vi "Read Theme.vi"(8 "error in":errorcluster, 11 "Popup in":refnum<class "Popup.lvclass">) -> (0 "error out":errorcluster, 2 "Theme.lvclass":refnum<class "Theme.lvclass">, 3 "Popup out":refnum<class "Popup.lvclass">)   [LabVIEW 2021, in "Pop-Up.lvlib" / "Popup.lvclass"]
doc: "Read the theme of the pop up\n\n<b>Code Developed By:</b> +\nDaniel Coons +\nhttps://github.com/danielcoons/tsc-pop-up"
uses:
  Popup.lvclass
  Theme/Theme.lvclass
  Popup.lvclass/Popup.ctl
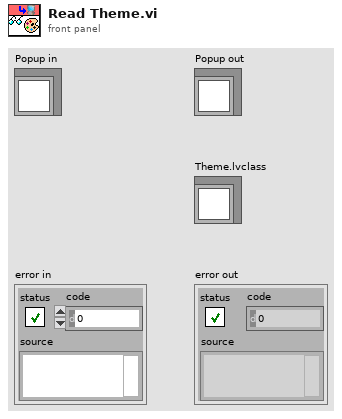
[diagram p1: front panel]
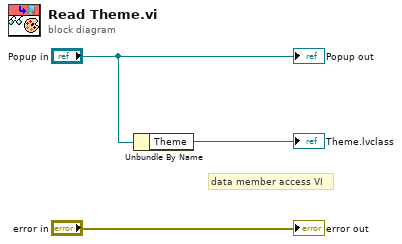
[diagram p0: block diagram]
diagram:
  # "data member access VI"
  n1 = Unbundle By Name("Popup in") -> ("Theme"=→"Theme.lvclass":refnum<class "Theme.lvclass">)
  "error out" <- "error in"
  "Popup out" <- "Popup in"
